vi "PXI-4130 Global Variable.vi"() -> ()   [LabVIEW 2009, in "PXI-4130 Custom Device.lvlib"]
uses:
  PXI-4130 Custom Device.lvlib
panel:
  in  "Continuous Read?":string="Continuous Read?"
  in  "Read Trigger":string="Read Trigger"
  in  "Channel #":string="Channel #"
  in  "Channel 1 Type":string="Channel 1 Type"
  in  "Channel 0 Type":string="Channel 0 Type"
  in  "Channel 1 Sense":string="Channel 1 Sense"
  in  "Channel 0 Sense":string="Channel 0 Sense"
  in  "Hardware Device Name":string="Hardware Device Name"
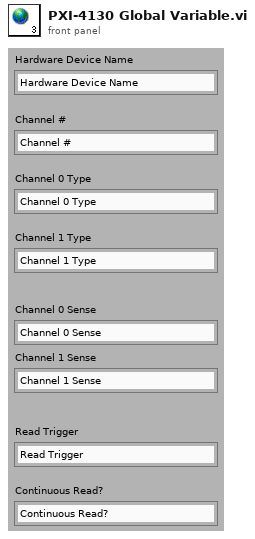
[diagram p1: front panel]
diagram:
